vi "GetTriggerMode.vi"(8 "Error In":errorcluster, 10 "Line (1-14)":u8=1 min=1 max=14 step=1, 11 "Kiethley 2602 In":refnum<visa-resource-name>) -> (0 "Error Out":errorcluster, 2 "Trigger Mode":T1, 3 "Keithley 2602 Out":refnum<visa-resource-name>)   [LabVIEW 2012, in "Keithley-2602.lvlib"]
uses:
  Keithley-2602.lvlib
  Controls/TriggerMode.ctl
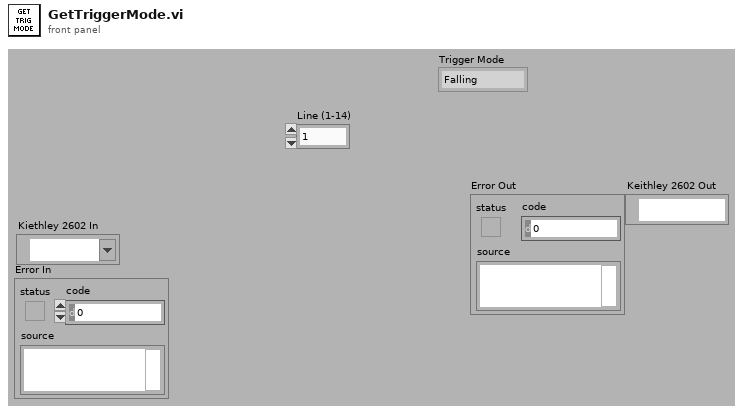
[diagram p1: front panel]
types:
  T1 = typedef "Keithley-2602.lvlib/TriggerMode.ctl" = enum16{"Falling", "Rising", "Either", "Synchronous"}
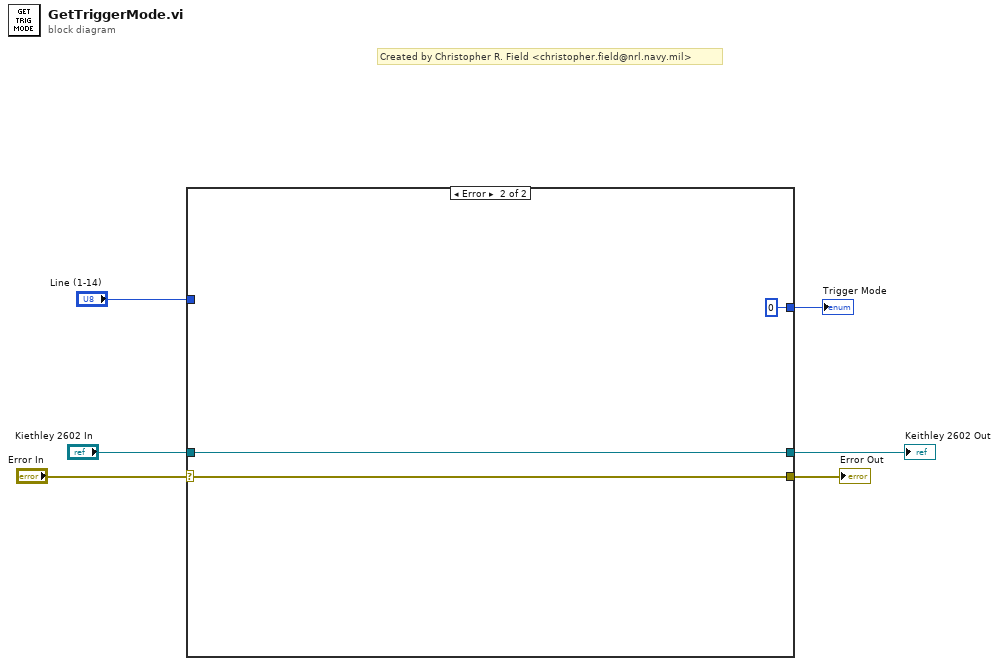
[diagram p0: block diagram]
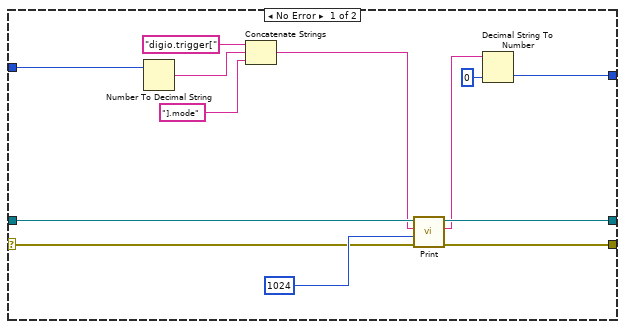
[diagram p2: hidden frame]
diagram:
  # "Created by Christopher R. Field <christopher.field@nrl.navy.mil>"
  n1 = case shown="Error" "Error In" {
    selector: "Error In" -> [w7 w21]
    tunnel: "Kiethley 2602 In" -> [w18 w22]
    tunnel: [w17 w22] -> w5
    tunnel: [w16 w21] -> w4
    tunnel: "Line (1-14)" -> [w14 _]
    tunnel: [w8 i16 0] -> w2
    frame No Error {
      n2 = Number To Decimal String(number=w14) -> (decimal integer string=w13:string)  [unwired: 1 in]
      n3 = Concatenate Strings("digio.trigger[", w13, "].mode") -> (w12:string)
      n4 = call "Print.vi"("Error In"=w7, "Byte Count"=u32 1024, "Attribute"=w12, "Kiethley 2602 In"=w18) -> ("Error Out"=w16:errorcluster, "Output"=w10:string, "Keithley 2602 Out"=w17:refnum<visa-resource-name>)  [unwired: 5 in]
      n5 = Decimal String To Number(string=w10, default (0L)=i16 0 ("default (0 I32)")) -> (number=w8:i16)  [unwired: 1 in, 1 out]
    }
    frame Error {
    }
  }
  "Error Out" <- w4
  "Keithley 2602 Out" <- w5
  "Trigger Mode" <- w2
